vi "stopcontar.vi"(8 "error in (no error)":errorcluster, 11 "ContadorB in":refnum<class "ContadorB.lvclass">) -> (0 "error out":errorcluster, 3 "ContadorB out":refnum<class "ContadorB.lvclass">)   [LabVIEW 2019, in "ContadorB.lvlib" / "ContadorB.lvclass"]
uses:
  ContadorB.lvclass
  ContadorB.lvclass/ContadorB.ctl
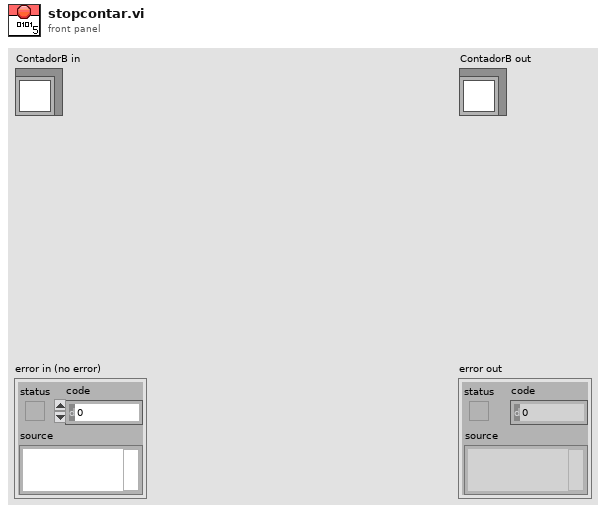
[diagram p1: front panel]
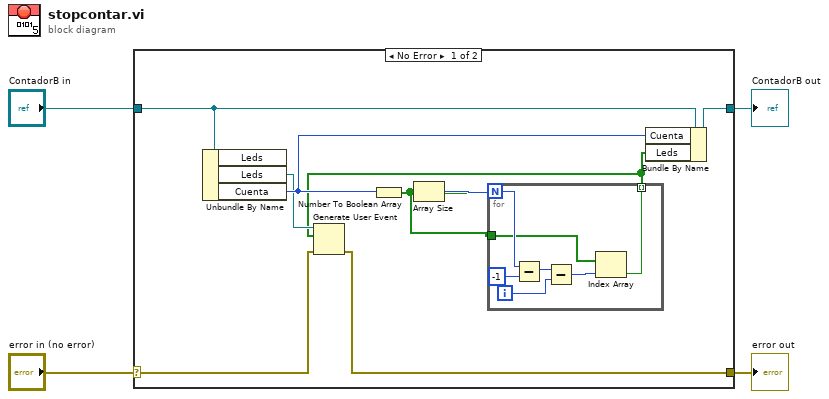
[diagram p0: block diagram]
diagram:
  n1 = case shown="No Error" "error in (no error)" {
    selector: "error in (no error)" -> [w7 w22]
    tunnel: [w6 w22] -> w3
    tunnel: [w11 w21] -> w1
    tunnel: "ContadorB in" -> [w13 w21]
    frame No Error {
      n2 = Unbundle By Name(w13) -> ("Leds"=w8:refnum<user-event>, "Cuenta"=w12:u8)  [unwired: 1 out]
      n3 = Number To Boolean Array(number=w12) -> (Boolean array=w9:bool[])
      n4 = Array Size(array=w9) -> (size(s)=w10:i32)
      n5 = for {
        N: w10 -> [w20]
        tunnel: w9 -> [w15]
        tunnel: [w14] -> w5 mode=indexing
        i -> [w17]
        n6 = Subtract(x=w20, y=-1) -> (x-y=w18:i32)
        n7 = Subtract(x=w18, y=w17) -> (x-y=w16:i32)
        n8 = Index Array(array=w15, index=w16) -> (element=w14:bool)
      }
      n9 = Generate User Event(user event=w8, event data cluster=w5, error in=w7) -> (error out=w6:errorcluster)  [unwired: 1 in, 1 out]
      n10 = Bundle By Name(cluster=w13, "Cuenta"=w12, "Leds"=w5) -> (w11:refnum<class "ContadorB.lvclass">)
    }
    frame Error {
    }
  }
  "error out" <- w3
  "ContadorB out" <- w1
